vi "Set Product Number.vi"(8 "error in (no error)":errorcluster caption="entrée d'erreur (pas d'erreur)", 10 "Product Number":string="STPH", 11 "Creation_SN_Nodon en entrée":refnum<class "Creation_SN_Nodon.lvclass">) -> (0 "error out":errorcluster caption="sortie d'erreur", 3 "Creation_SN_Nodon en sortie":refnum<class "Creation_SN_Nodon.lvclass">)   [LabVIEW 2020, in "Library Instrument & Equipement.lvlib" / "Library Creation_SN.lvlib" / "Creation_SN_Nodon.lvclass"]
uses:
  Creation_SN_Nodon.lvclass
  Creation_SN_Nodon.lvclass/Creation_SN_Nodon.ctl
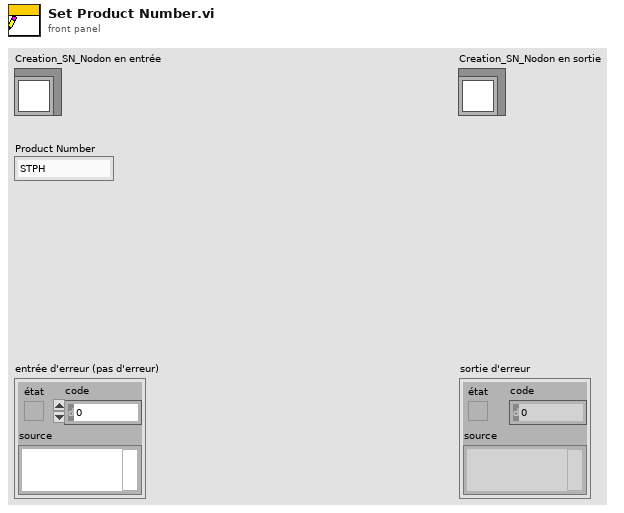
[diagram p1: front panel]
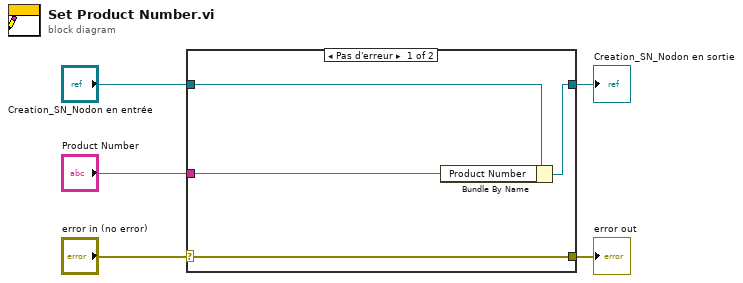
[diagram p0: block diagram]
diagram:
  n1 = case shown="Pas d'erreur" "error in (no error)" {
    selector: "error in (no error)" -> [w9 w10]
    tunnel: [w9 w10] -> w4
    tunnel: [w7 w11] -> w2
    tunnel: "Creation_SN_Nodon en entrée" -> [w8 w11]
    tunnel: "Product Number" -> [w6 _]
    frame No Error {
      n2 = Bundle By Name(cluster=w8, "Product Number"=w6) -> (w7:refnum<class "Creation_SN_Nodon.lvclass">)
    }
    frame Error {
    }
  }
  "error out" <- w4
  "Creation_SN_Nodon en sortie" <- w2
